vi "CLSUIP_ReplaceClassCtls.vi"(4 "error in (no error)":errorcluster, 7 "VIRetooler":refnum<class "VIRetooler.lvclass">) -> (0 "error out":errorcluster, 3 "VIRetooler out":refnum<class "VIRetooler.lvclass">)   [LabVIEW 2021, in "MemberVICreation.lvlib" / "VIRetooler.lvclass"]
uses:
  <resource>/Framework/Providers/LVClassLibrary/NewAccessors/VIRetooler/VIRetooler.lvclass
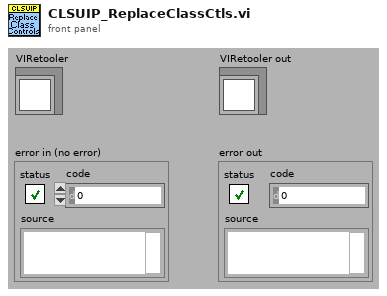
[diagram p1: front panel]
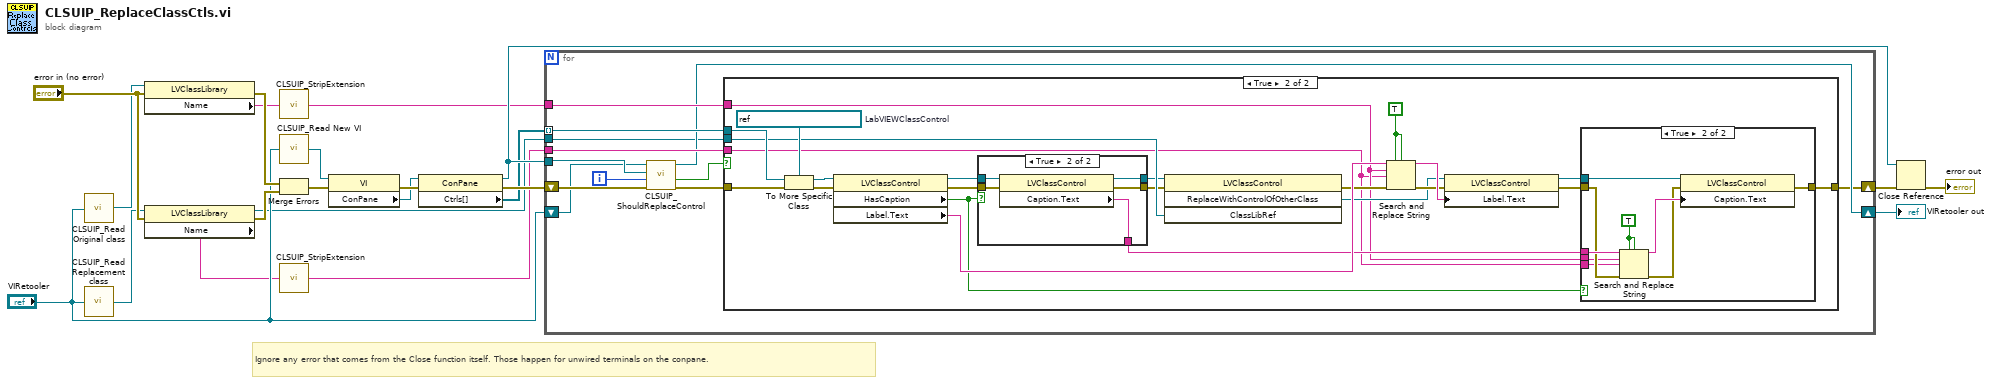
[diagram p0: block diagram]
diagram:
  # "Ignore any error that comes from the Close function itself. Those happen for unwired terminals on the conpane."
  n1 = call <resource>:"CLSUIP_Read Original class.vi"("VIRetooler.lvclass in"="VIRetooler") -> ("Orig class"=w7:refnum<vi>)
  n2 = call <resource>:"CLSUIP_Read Replacement class.vi"("VIRetooler.lvclass in"="VIRetooler") -> ("Replacement class"=w6:refnum<vi>)
  n3 = property class="LVClassLibrary"(reference=w7, error in="error in (no error)") -> (error out=w13:errorcluster, "Name"=w4:string)  [unwired: 1 out]
  n4 = property class="LVClassLibrary"(reference=w6, error in="error in (no error)") -> (reference out=w1:refnum<vi>, error out=w12:errorcluster, "Name"=w3:string)
  n5 = call <resource>:"CLSUIP_StripExtension.vi"("string"=w4) -> ("string without extension"=w10:string)
  n6 = call <resource>:"CLSUIP_Read New VI.vi"("VIRetooler.lvclass in"="VIRetooler") -> ("New VI"=w8:refnum<vi>)
  n7 = Merge Errors(w13, w12) -> (w11:errorcluster)
  n8 = call <resource>:"CLSUIP_StripExtension.vi"("string"=w3) -> ("string without extension"=w9:string)
  n9 = property class="VI"(reference=w8, error in=w11) -> (error out=w16:errorcluster, "ConPane"=w15:refnum<vi>)  [unwired: 1 out]
  n10 = property class="ConPane"(reference=w15, error in=w16) -> (reference out=w20:refnum<vi>, error out=w18:errorcluster, "Ctrls[]"=w17:refnum<vi>[])
  n11 = for {
    tunnel: w17 -> [w29] mode=indexing
    shift-right: [w23] -> w19
    shift-left: w18 -> [w31]
    tunnel: w20 -> [w33]
    tunnel: w10 -> [w27]
    tunnel: w9 -> [w26]
    shift-right: [w24] -> w2
    shift-left: "VIRetooler" -> [w25]
    tunnel: w1 -> [w22]
    i -> [w32]
    n12 = call-dynamic "CLSUIP_ShouldReplaceControl.vi"("error in (no error)"=w31, "Terminal Index"=w32, "ConPane"=w33, "VIRetooler"=w25) -> ("error out"=w28:errorcluster, "Should replace?"=w30:bool, "VIRetooler 2"=w24:refnum<class "VIRetooler.lvclass">)  [unwired: 1 out]
    n13 = case shown="True" w30 {
      tunnel: w29 -> [_ w53]
      tunnel: w28 -> [w34 w51]
      tunnel: [w34 w39] -> w23
      tunnel: w27 -> [_ w36]
      tunnel: w26 -> [_ w35]
      tunnel: w22 -> [_ w49]
      frame False {
      }
      frame True {
        w54 = refnum<vi> refnum  # LabVIEWClassControl
        w56 = TRUE ("replace all? (F)")
        n14 = To More Specific Class(target class=w54, reference=w53, error in=w51) -> (specific class reference=w52:refnum<vi>, error out=w50:errorcluster)
        n15 = property class="LVClassControl"(reference=w52, error in=w50) -> (reference out=w46:refnum<vi>, error out=w45:errorcluster, "HasCaption"=w38:bool, "Label.Text"=w57:string)
        n16 = case shown="True" w38 {
          tunnel: [w69 w72] -> w47
          tunnel: w46 -> [w69 w74]
          tunnel: [w68 w71] -> w44
          tunnel: w45 -> [w68 w73]
          tunnel: [_ w70] -> w37
          frame False {
          }
          frame True {
            n17 = property class="LVClassControl"(reference=w74, error in=w73) -> (reference out=w72:refnum<vi>, error out=w71:errorcluster, "Caption.Text"=w70:string)
          }
        }
        n18 = invoke class="LVClassControl" method="ReplaceWithControlOfOtherClass"(reference=w47, error in=w44, "ClassLibRef"=w49) -> (error out=w48:errorcluster, "ReplaceWithControlOfOtherClass"=w42:refnum<vi>)  [unwired: 1 in, 2 out]
        n19 = Search and Replace String(replace all?=w56, case sensitive?=w56, input string=w57, search string=w36, replace string=w35, error in=w48) -> (result string=w55:string, error out=w43:errorcluster)  [unwired: 4 out]
        n20 = property class="LVClassControl"(reference=w42, error in=w43, "Label.Text"=w55) -> (reference out=w41:refnum<vi>, error out=w40:errorcluster)
        n21 = case shown="True" w38 {
          tunnel: w41 -> [_ w67]
          tunnel: w40 -> [w58 w62]
          tunnel: [w58 w66] -> w39
          tunnel: w37 -> [_ w64]
          tunnel: w36 -> [_ w60]
          tunnel: w35 -> [_ w59]
          frame False {
          }
          frame True {
            w65 = TRUE ("replace all? (F)")
            n22 = Search and Replace String(replace all?=w65, case sensitive?=w65, input string=w64, search string=w60, replace string=w59, error in=w62) -> (result string=w63:string, error out=w61:errorcluster)  [unwired: 4 out]
            n23 = property class="LVClassControl"(reference=w67, error in=w61, "Caption.Text"=w63) -> (error out=w66:errorcluster)  [unwired: 1 out]
          }
        }
      }
    }
  }
  "VIRetooler out" <- w2
  n24 = Close Reference(reference=w20, error in (no error)=w19) -> (error out=→"error out":errorcluster)
